vi "ois_ttc_merging.vi"() -> ()   [LabVIEW 2012]
uses:
  <vilib>/vision/Image Controls.llb/IMAQ Image.ctl
  <vilib>/picture/picture.llb/imagedata.ctl
  <vilib>/Utility/file.llb/Write To Spreadsheet File (DBL).vi
  <vilib>/vision/NI_Vision_Development_Module.lvlib
panel:
  in  "Tab Control":T1(tab)
  out "avi image with mask":T2(plugin-control)
  in  "video file":path=path "\\\\IFMB-02-024B-10\\Ischemia2/OOS/2019-05-29/2019-05-29_11-14-53.avi"
  in  "Use mask":bool=TRUE
  out "avi image":T2(plugin-control)
  in  "Range":cluster{"Lower value":sgl, "Upper value":sgl}={"Lower value"=103.29114, "Upper value"=255.0} {"Upper value" scale=0.0..255.0; "Lower value" scale=0.0..255.0}
  in  "IOS color":u32(colorbox)=16860
  in  "line color":u32(colorbox)=16711680
  in  "line Width":u32=1
  in  "TTC file":path=path "D:/Neurolab/ialdev/Ischemia YG/analisys/TTC images and OIS comparison/template/cortex_ttc_template.tif"
  in  "TTC Angle":dbl(knob) caption="Angle"
  in  "TTC Zoom":dbl(slide)=0.23059004545211792 caption="Zoom" scale=0.001..1.0
  in  "center X":u32(slide)=640 scale=0.0..640.0
  in  "center Y":u32(slide)=471
  in  "TTC horizontal reverse":bool caption="Horizontal reverse"
  in  "TTC vertical reverse":bool caption="Vertical reverse"
  out "front TTC image 2":T2(plugin-control) caption="TTC image"
  in  "Clear all points":bool
  out "XY Graph":cluster{dbl[], dbl[]}[](graph) caption="Saturation"
  in  "Add point":bool
  in  "Delete last point":bool
  in  "Save All Data":bool
  in  "filename":string="2019-05-29_11-14-53"
  in  "base path":path=path "\\\\IFMB-02-024B-10\\Ischemia2/OOS/2019-05-29"
  out "settings file":path=path "D:/Neurolab/ialdev/Ischemia YG/analisys/TTC images and OIS comparison/settings.ini"
  in  "Kernel Size (3,5,...)":i32=5 min=3 step=2
  in  "filtering":i32=5 min=0 max=100
  out "error out 2":errorcluster
  out "IOS borders and avi image":T3(array[cluster])
  out "ttc color on borders":cluster{"Slide":dbl, u32[]}[](array[cluster])
  out "IOS borders":u8[][](array[numeric])
  out "Array":dbl[](array[numeric])=[393.78881454467773, 286.3416109085083, 886.2111854553223, 655.6583890914917]
  out "ttc image data":T4={"image type"=0, "image depth"=24, "image"=array[143172 elements], "mask"=[], "colors"=[], "Rectangle"={"left"=0, "top"=0, "right"=246, "bottom"=194}}
  out "ios overlay":u32[][](array[numeric])
  out "error out 4":errorcluster
  out "dt":u32=2500
  in  "Time, min":dbl(slide)=2.057065217391304 scale=0.0..2.375
  out "error out":errorcluster
  out "TTC image in":T2
  in  "stop":bool=TRUE
  out "front TTC image":T2(plugin-control)
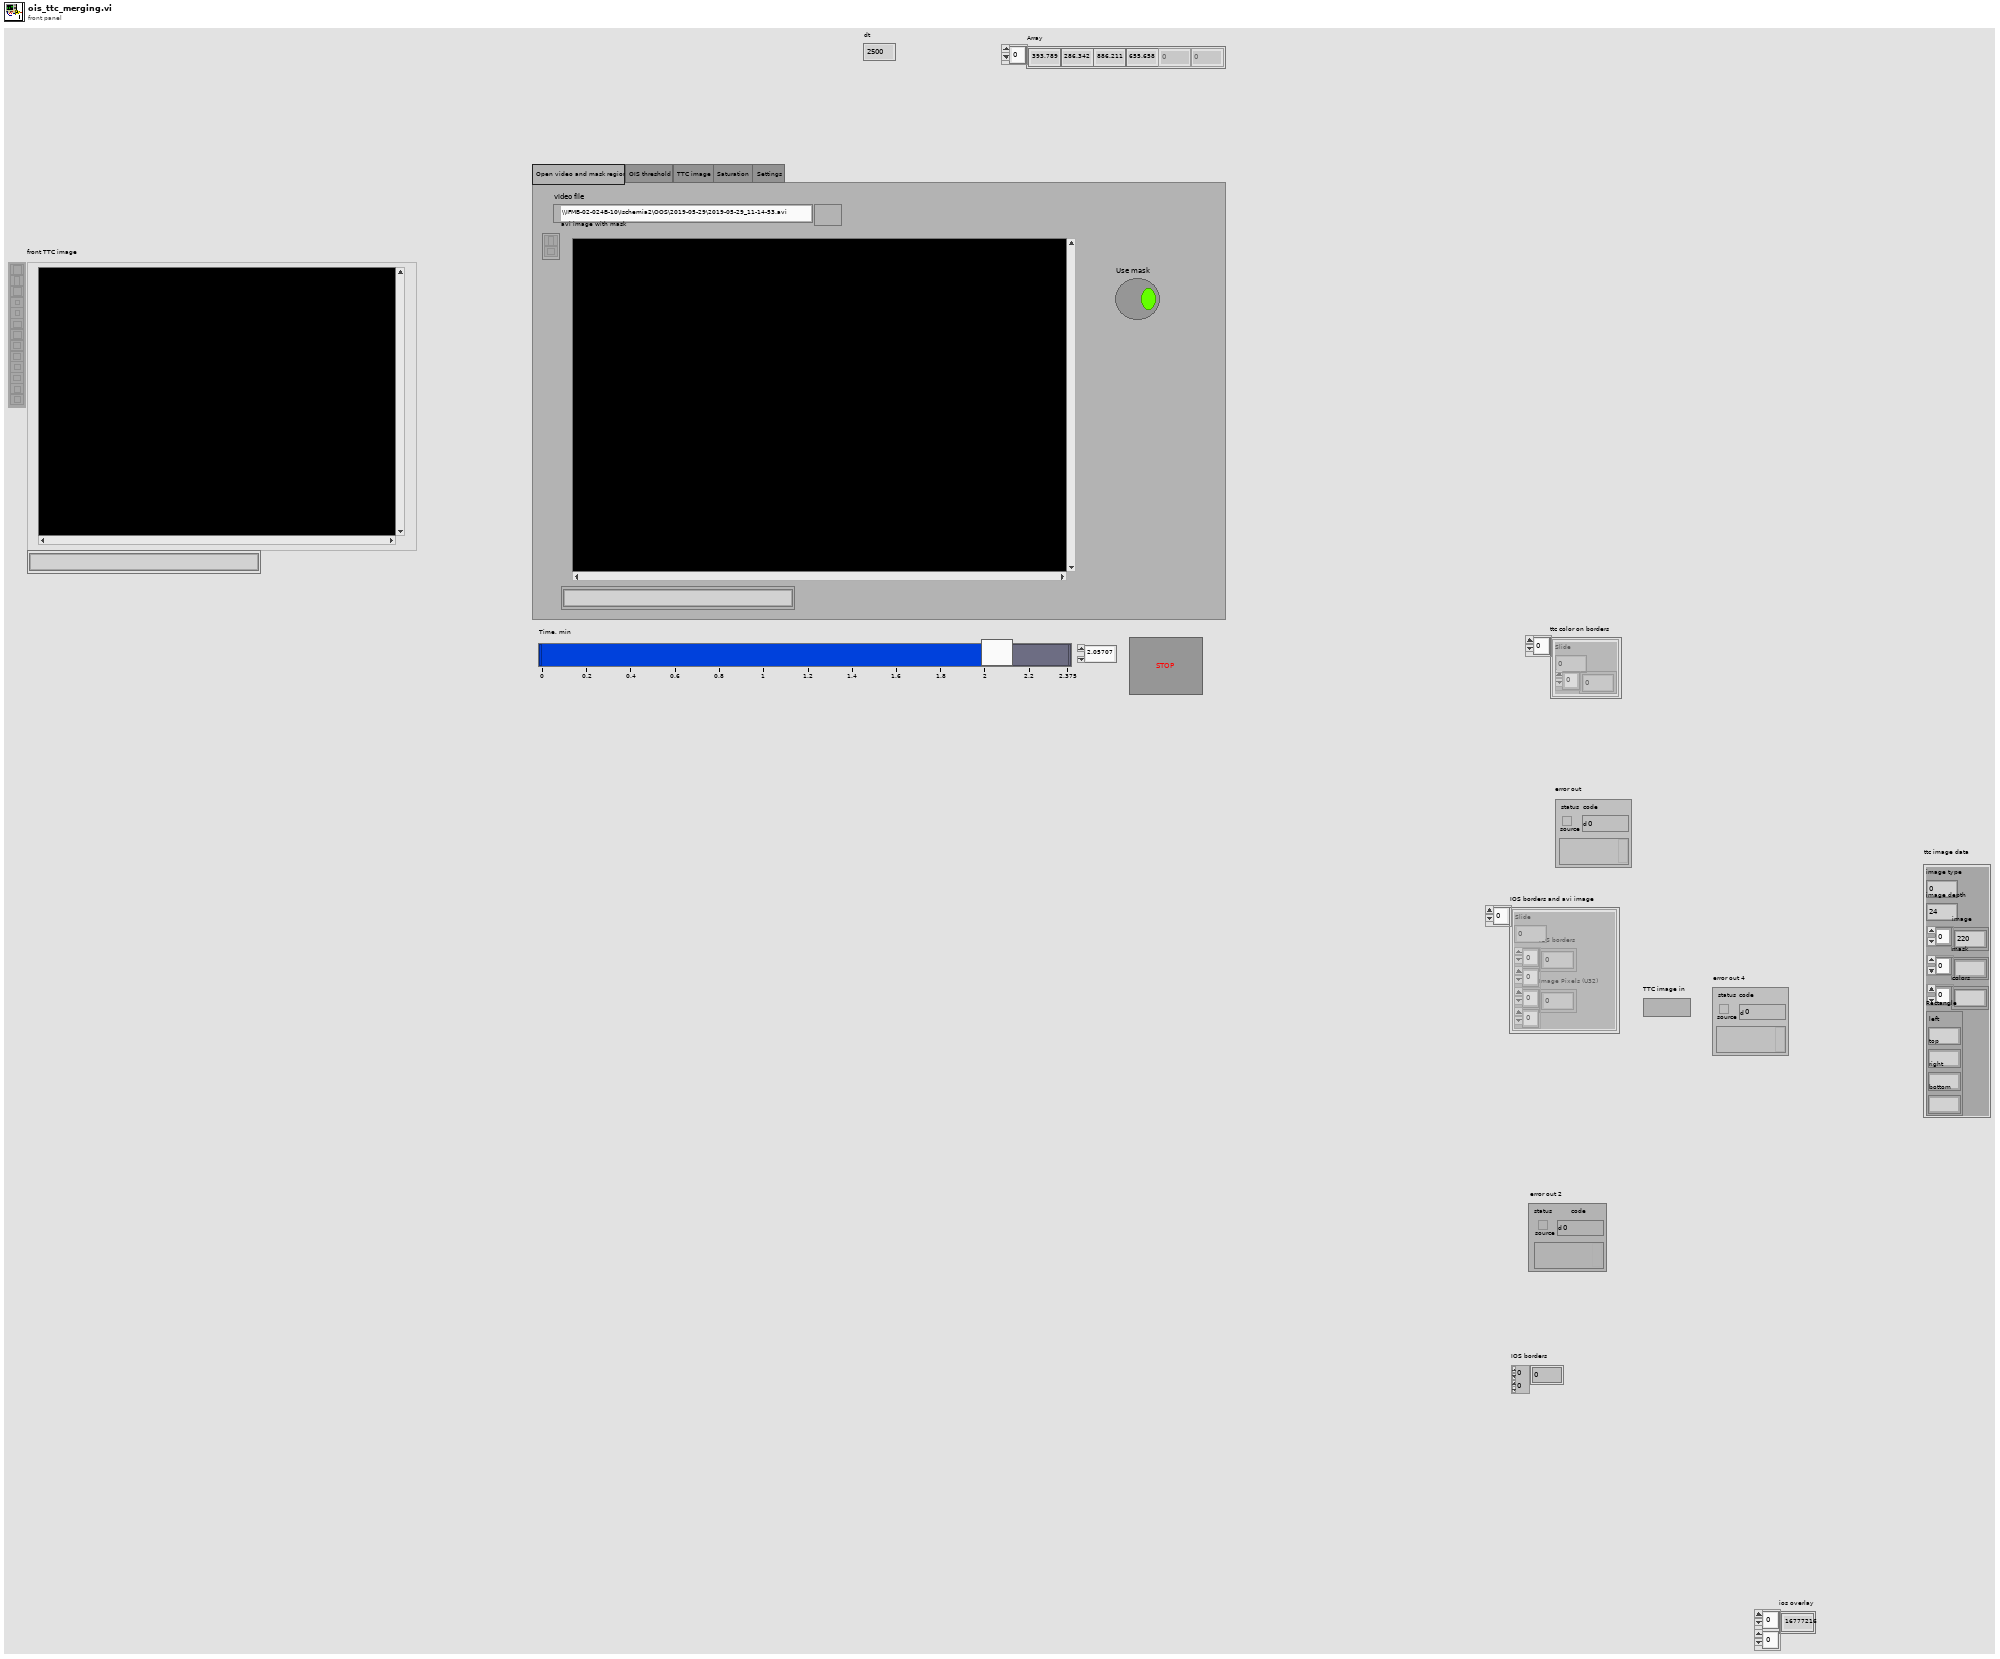
[diagram p1: front panel]
types:
  T1 = enum32{"Open video and mask region", "OIS threshold", "TTC image", "Saturation", "Settings"}
  T2 = typedef "IMAQ Image.ctl" = refnum<image>
  T3 = cluster{"Slide":dbl, "IOS borders":u8[][], "Image Pixels (U32)":u32[][]}[]
  T4 = typedef "imagedata.ctl" = cluster{"image type":i32, "image depth":i32, "image":u8[], "mask":u8[], "colors":u32[], "Rectangle":cluster{"left":i16, "top":i16, "right":i16, "bottom":i16}}
  T5 = typedef "Image Type" = u32
  T6 = enum16{"open", "replace", "create", "open or create", "replace or create", "replace or create with confirmation"}
  T7 = typedef "AviRefnum.ctl" = refnum<k1>
  T8 = cluster{"Range":cluster{"Lower value":sgl, "Upper value":sgl}, "IOS color":u32, "line color":u32, "line Width":u32}
  T9 = enum32{"AutoM", "Close", "Dilate", "Erode", "Gradient", "Gradient out", "Gradient in", "Hit miss", "Open", "PClose", "POpen", "Thick", "Thin"}
  T10 = cluster{"Global Rectangle":i32[], "Contours":cluster{"Contour Type":u32, "ROI Type":u32, "Points":i32[]}[]}
  T11 = cluster{"Time, min":dbl, "IOS borders":u8[][], "Image Pixels (U32)":u32[][]}
  T12 = cluster{"video file":path, "TTC file":path, "TTC Angle":dbl, "TTC Zoom":dbl, "center X":u32, "center Y":u32, "TTC horizontal reverse":bool, "TTC vertical reverse":bool, "ROI":cluster{"Global Rectangle":i32[], "Contours":cluster{"Contour Type":u32, "ROI Type":u32, "Points":i32[]}[]}, "Range":cluster{"Lower value":sgl, "Upper value":sgl}, "Image Pixels (U32)":u32[][], "ttc color on borders":cluster{"Slide":dbl, u32[]}[], "IOS borders and avi image":cluster{"Slide":dbl, "IOS borders":u8[][], "Image Pixels (U32)":u32[][]}[]}
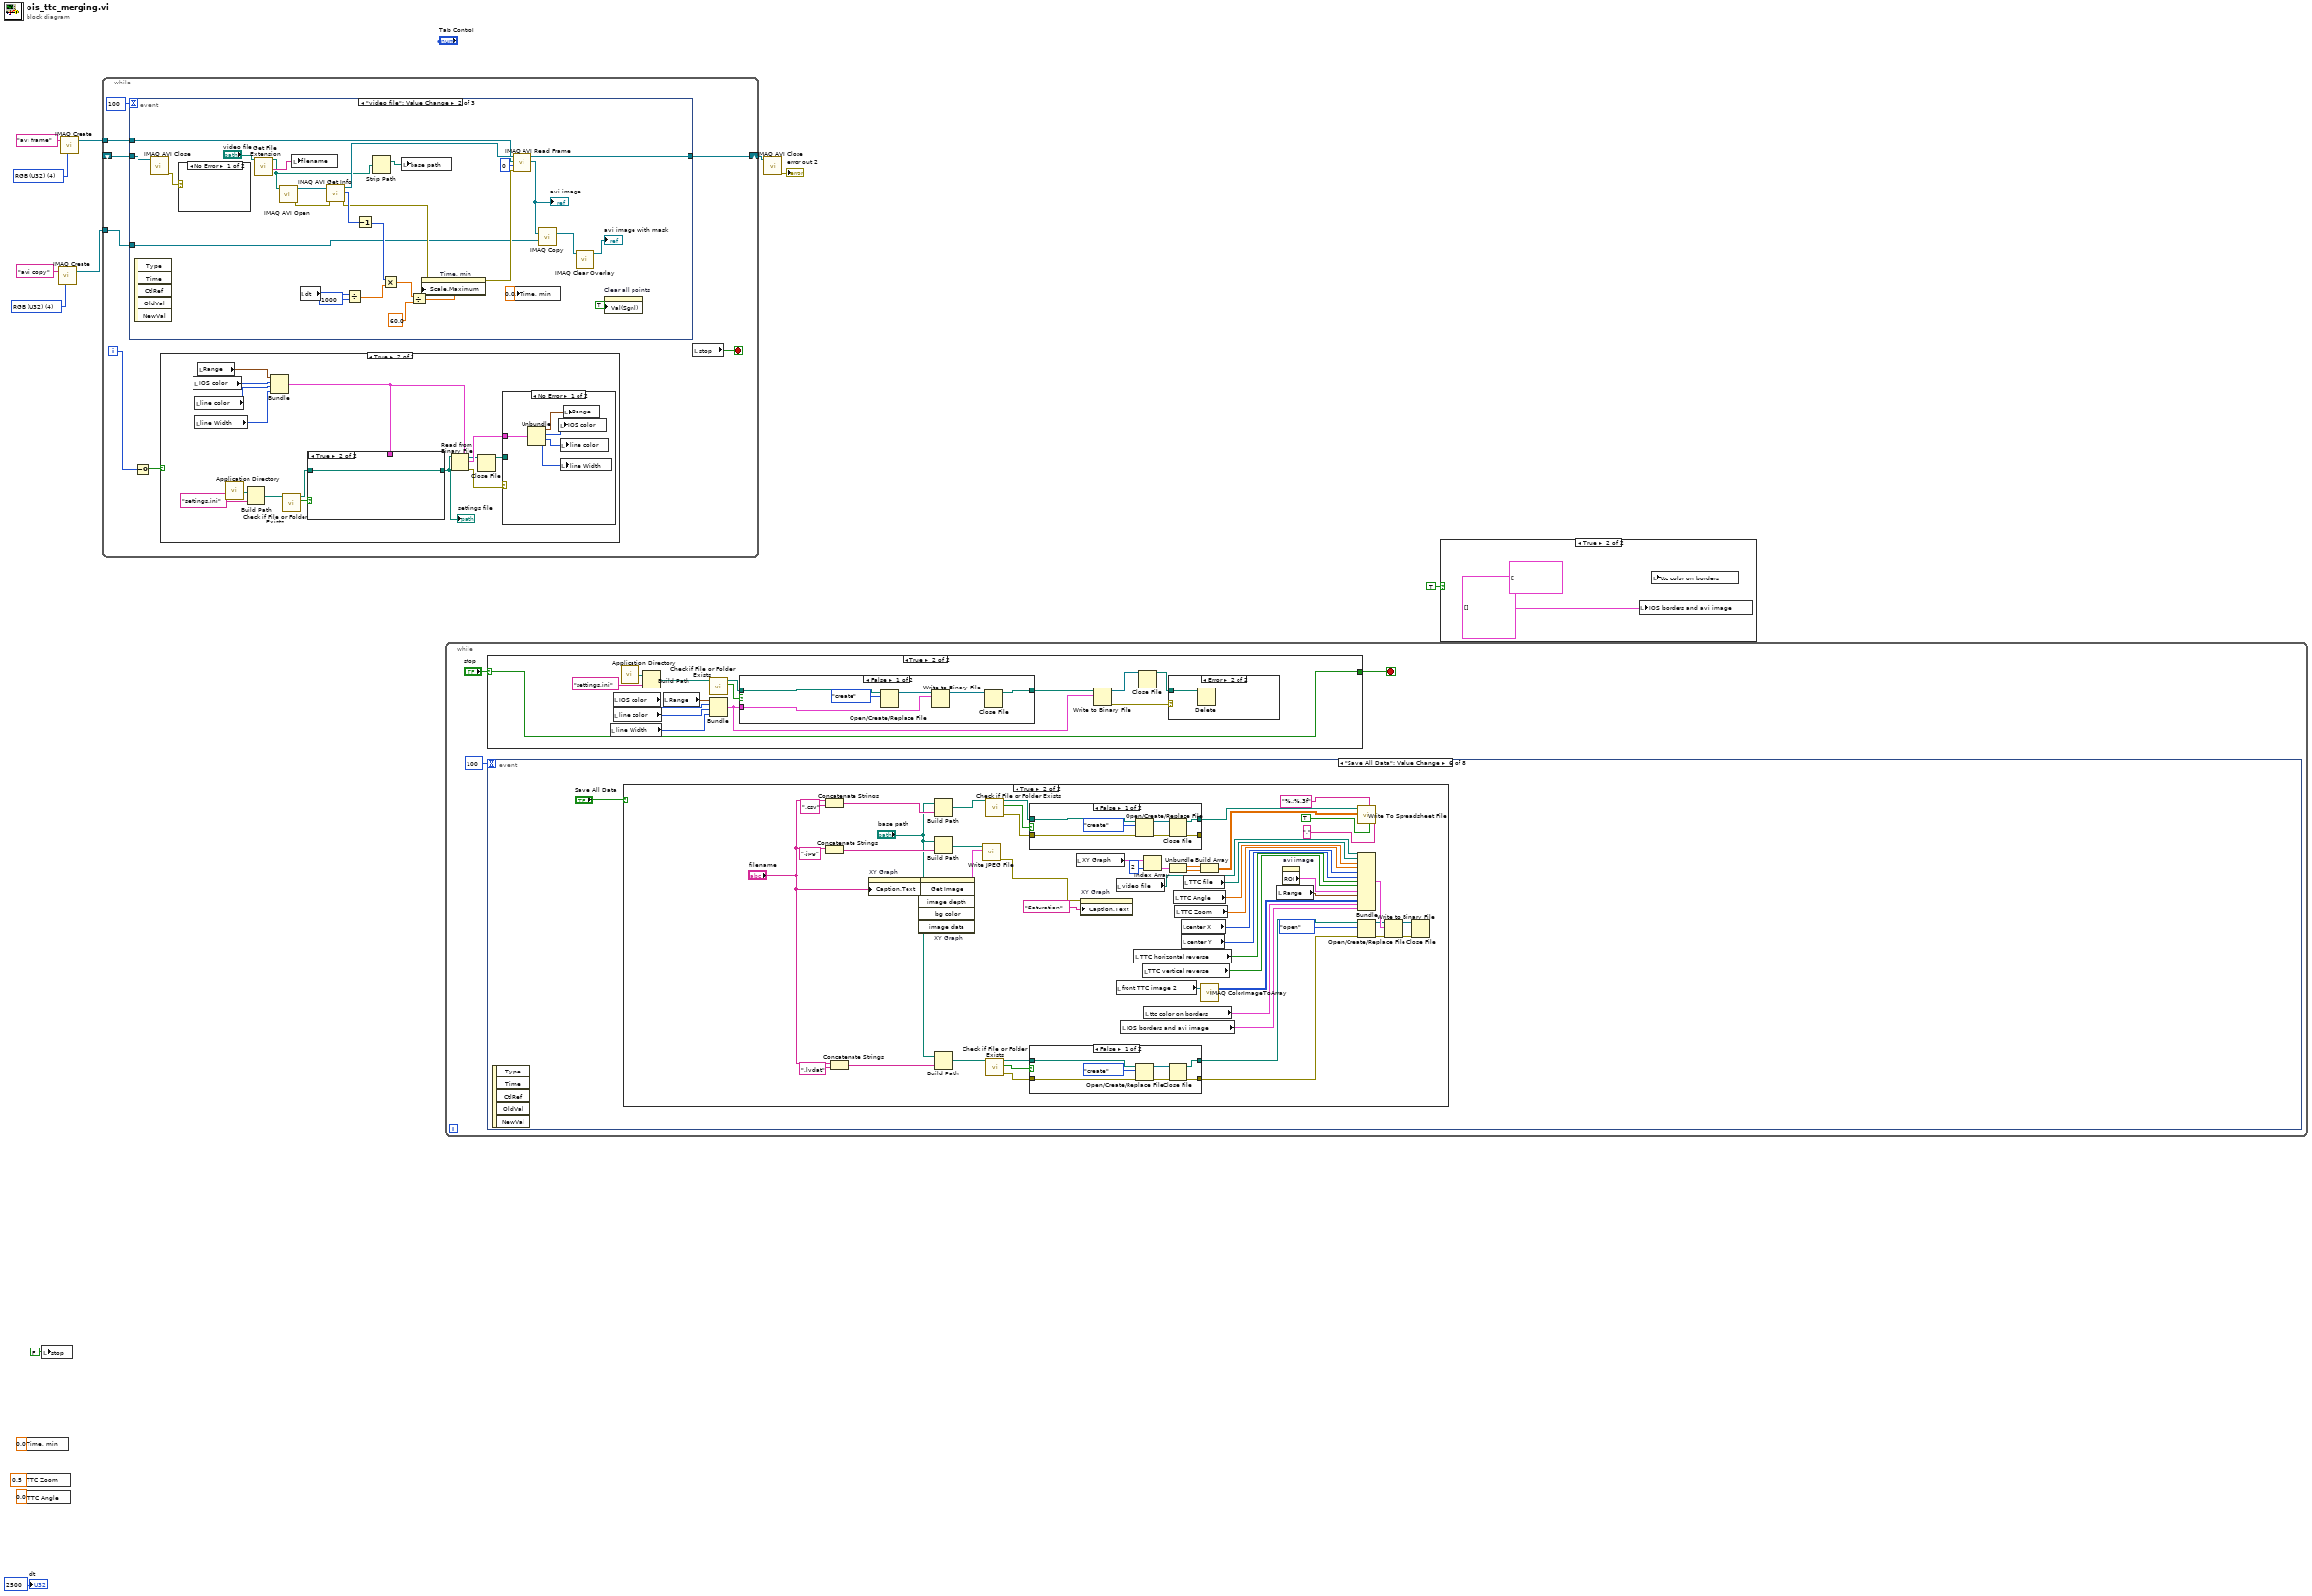
[diagram p0: block diagram]
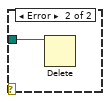
[diagram p4: hidden frame]
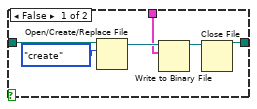
[diagram p5: hidden frame]
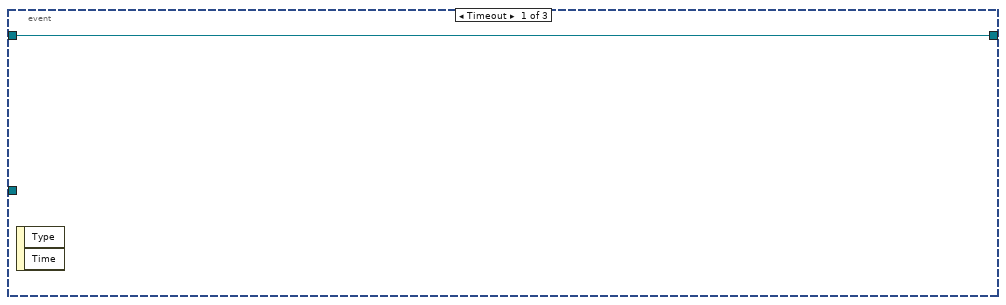
[diagram p6: hidden frame]
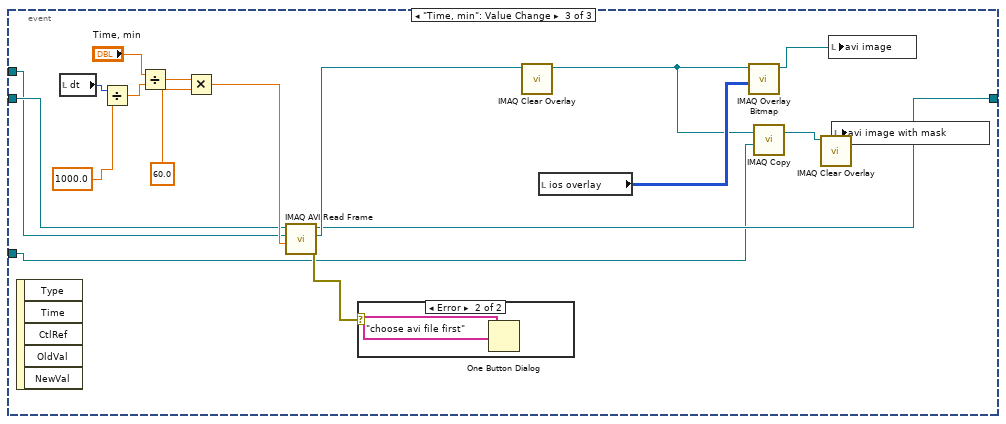
[diagram p8: hidden frame]
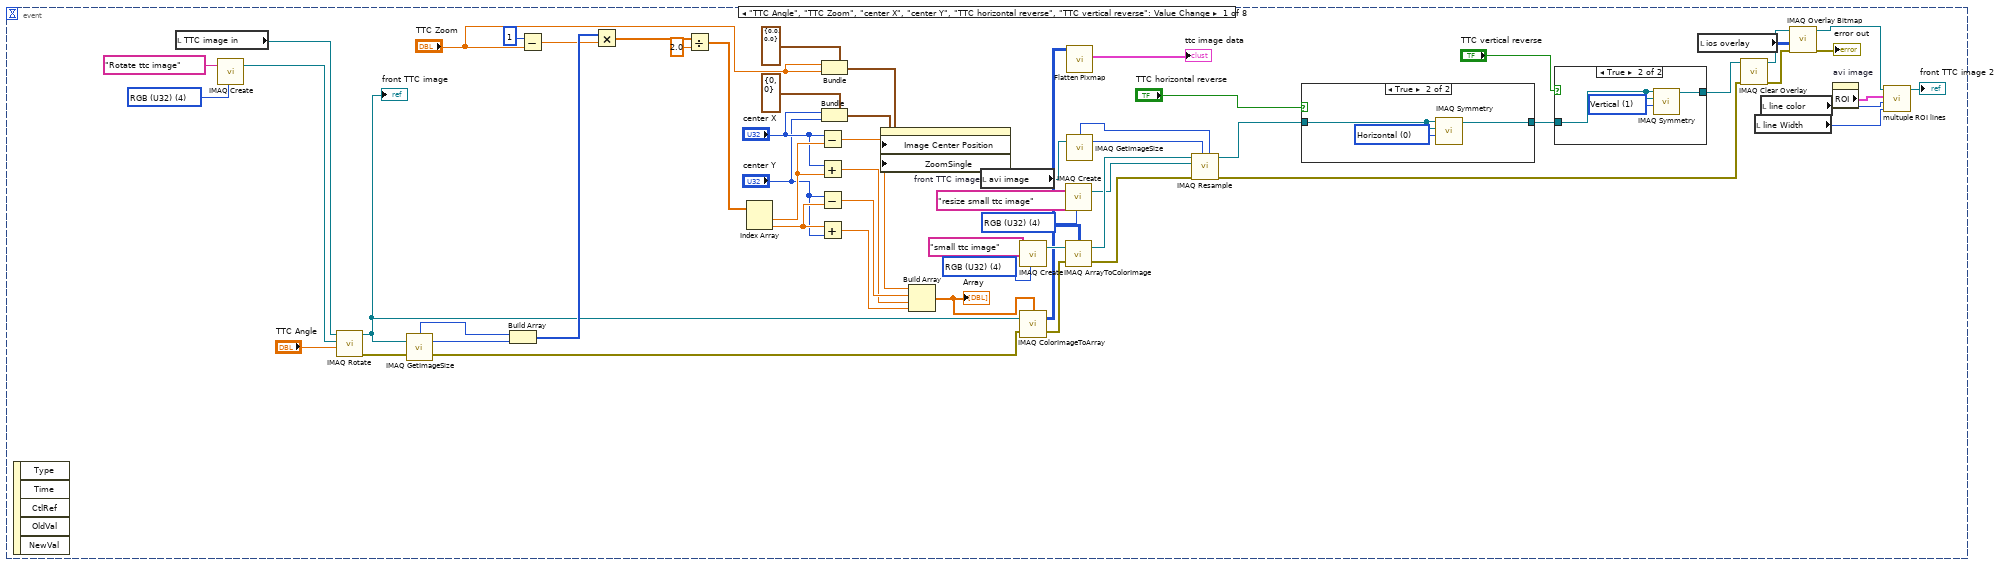
[diagram p13: hidden frame]
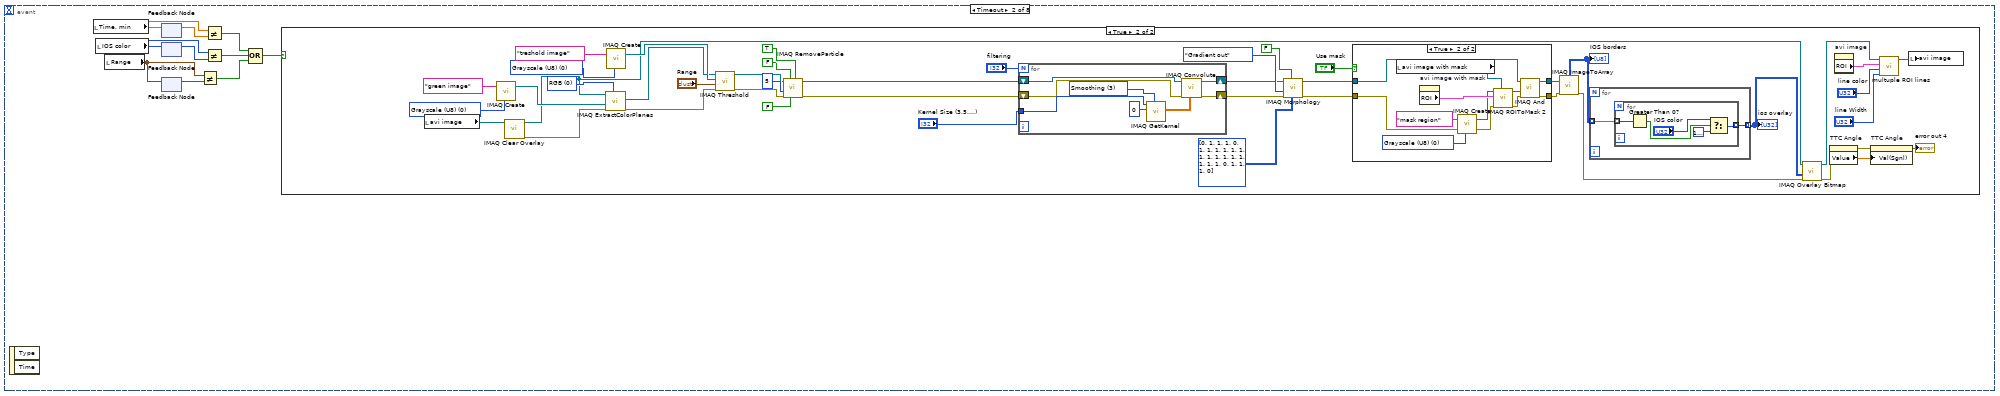
[diagram p16: hidden frame]
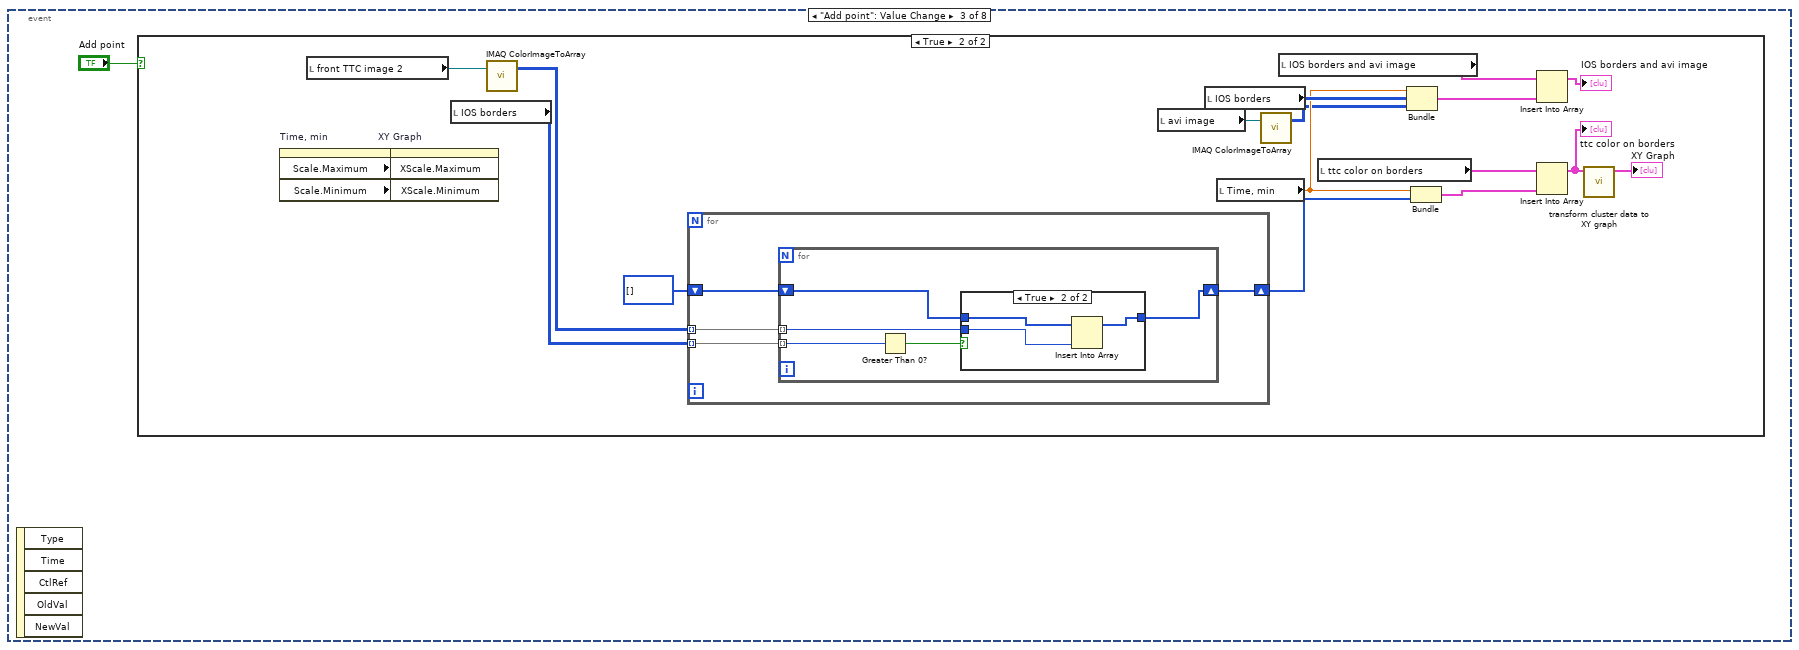
[diagram p19: hidden frame]
diagram:
  w2 = T5 4 items=["Grayscale (U8)", "Grayscale (I16)", "Grayscale (SGL)", "Complex (CSG)", "RGB (U32)", "HSL (U32)", "RGB (U64)", "Grayscale (U16)"] ("Image Type")
  w9 = T5 4 items=["Grayscale (U8)", "Grayscale (I16)", "Grayscale (SGL)", "Complex (CSG)", "RGB (U32)", "HSL (U32)", "RGB (U64)", "Grayscale (U16)"] ("Image Type")
  n1 = local write "Time, min"(0.0 ("Slide")) -> ()
  n2 = local write "TTC Zoom"(0.5 ("Zoom")) -> ()
  n3 = local write "TTC Angle"(0.0 ("Slide")) -> ()
  n4 = local write "stop"(FALSE ("stop")) -> ()
  n5 = call "IMAQ Create"("Image Name"="avi copy", "Image Type"=w2) -> ("New Image"=w1:T2)  [unwired: 3 in, 1 out]
  n6 = call "IMAQ Create"("Image Name"="avi frame", "Image Type"=w9) -> ("New Image"=w7:T2)  [unwired: 3 in, 1 out]
  n7 = while {
    shift-right: [w20] -> w6
    shift-left: _ -> [w18]
    tunnel: w7 -> [w19]
    tunnel: w1 -> [w17]
    i -> [w15]
    stop <- w22 stop-if-true
    n8 = event shown="[1] \"video file\": Value Change" {
      selector: _ -> [_ _ _]
      dyn-events: _ -> [_ _ _]
      timeout: 100 -> [_ _ _]
      tunnel: [w51 w64 w86] -> w20
      tunnel: w19 -> [_ w63 w84]
      tunnel: w18 -> [w51 w62 w85]
      tunnel: w17 -> [_ w58 w82]
      event Timeout {
        n9 = event-data() -> ()  [unwired: 1 in, 2 out]
      }
      event "video file": Value Change {
        n10 = event-data() -> ()  [unwired: 1 in, 5 out]
        n11 = call "IMAQ AVI Close"("Avi Refnum"=w62) -> ("error out"=w61:errorcluster)  [unwired: 10 in]
        n12 = case shown="No Error" w61 {
          frame No Error {
          }
          frame Error {
          }
        }
        n13 = call <vilib>:"Get File Extension.vi"("file"="video file") -> ("filename without extension"=w54:string, "dup file"=w53:path)  [unwired: 7 in, 2 out]
        n14 = call "IMAQ AVI Open"("AVI Path"=w53) -> ("error out"=w67:errorcluster, "Avi Refnum"=w79:T7)  [unwired: 9 in]
        n15 = local write "filename"(w54) -> ()
        n16 = local read "dt"() -> (w74:u32)
        n17 = call "IMAQ AVI Get Info"("error in (no error)"=w67, "Avi Refnum"=w79) -> ("error out"=w66:errorcluster, "Number of Frames"=w77:u32, "Avi Refnum (duplicate)"=w78:T7)  [unwired: 5 in, 2 out]
        n18 = Divide(x=w74, y=u32 1000) -> (x/y=w71:dbl)
        n19 = Decrement(x=w77) -> (x-1=w72:u32)
        n20 = Strip Path(path=w53) -> (stripped path=w52:path)  [unwired: 1 out]
        n21 = Multiply(x=w72, y=w71) -> (x*y=w70:dbl)
        n22 = local write "base path"(w52) -> ()
        n23 = Divide(x=w70, y=60.0) -> (x/y=w68:dbl)
        n24 = property on="Time, min" class="Slide (strict)"(error in=w66, "Scale.Maximum"=w68) -> (error out=w65:errorcluster)  [unwired: 1 in, 1 out]
        n25 = local write "Time, min"(0.0 ("Slide")) -> ()
        n26 = call "IMAQ AVI Read Frame"("error in (no error)"=w65, "Frame Number"=u32 0, "Image"=w63, "Avi Refnum"=w78) -> ("Image Out"=w59:T2, "Avi Refnum (duplicate)"=w64:T7)  [unwired: 4 in, 2 out]
        "avi image" <- w59
        n27 = call "IMAQ Copy"("Image Dst"=w58, "Image Src"=w59) -> ("Image Dst Out"=w57:T2)  [unwired: 4 in, 1 out]
        n28 = call "IMAQ Clear Overlay"("Image"=w57) -> ("Image Out"=→"avi image with mask":T2)  [unwired: 9 in, 1 out]
        n29 = property on="Clear all points" class="Bool (strict)"("Val(Sgnl)"=TRUE ("Value (Signaling)")) -> ()  [unwired: 2 in, 2 out]
      }
      event "Time, min": Value Change {
        n30 = event-data() -> ()  [unwired: 1 in, 5 out]
        n31 = local read "dt"() -> (w96:u32)
        n32 = Divide(x=w96, y=1000.0) -> (x/y=w93:dbl)
        n33 = Divide(x="Time, min", y=w93) -> (x/y=w92:dbl)
        n34 = Multiply(x=w92, y=60.0) -> (x*y=w90:dbl)
        n35 = call "IMAQ AVI Read Frame"("Frame Number"=w90, "Image"=w84, "Avi Refnum"=w85) -> ("error out"=w97:errorcluster, "Image Out"=w88:T2, "Avi Refnum (duplicate)"=w86:T7)  [unwired: 5 in, 1 out]
        n36 = case shown="Error" w97 {
          frame No Error {
          }
          frame Error {
            n37 = One Button Dialog(message="choose avi file first") -> ()  [unwired: 1 in, 1 out]
          }
        }
        n38 = call "IMAQ Clear Overlay"("Image"=w88) -> ("Image Out"=w81:T2)  [unwired: 9 in, 1 out]
        n39 = local read "ios overlay"() -> (w87:u32[][])
        n40 = call "IMAQ Overlay Bitmap"("Bitmap"=w87, "Image"=w81) -> ("Image Out"=w89:T2)  [unwired: 8 in, 1 out]
        n41 = call "IMAQ Copy"("Image Dst"=w82, "Image Src"=w81) -> ("Image Dst Out"=w83:T2)  [unwired: 4 in, 1 out]
        n42 = call "IMAQ Clear Overlay"("Image"=w83) -> ("Image Out"=w80:T2)  [unwired: 9 in, 1 out]
        n43 = local write "avi image"(w89) -> ()
        n44 = local write "avi image with mask"(w80) -> ()
      }
    }
    n45 = Equal To 0?(x=w15) -> (x = 0?=w16:bool)
    n46 = case shown="True" w16 {
      frame False {
      }
      frame True {
        n47 = local read "IOS color"() -> (w30:u32)
        n48 = local read "line color"() -> (w28:u32)
        n49 = local read "line Width"() -> (w29:u32)
        n50 = local read "Range"() -> (w31:cluster{"Lower value":sgl, "Upper value":sgl})
        n51 = call <vilib>:"Application Directory.vi"() -> ("Application Directory"=w37:path)
        n52 = Build Path(base path=w37, name or relative path="settings.ini") -> (appended path=w34:path)
        n53 = Bundle("Range"=w31, "IOS color"=w30, "line color"=w28, "line Width"=w29) -> (w27:T8)  [unwired: 1 in]
        n54 = call <vilib>:"Check if File or Folder Exists.vi"("path"=w34) -> ("file or folder exists?"=w35:bool, "dup path"=w36:path)  [unwired: 8 in, 1 out]
        n55 = case shown="True" w35 {
          tunnel: w36 -> [w49 w50]
          tunnel: [w44 w50] -> w32
          tunnel: w27 -> [w45 _]
          frame False {
            n56 = Open/Create/Replace File(file path (use dialog)=w49, operation (0:open)=T6."create") -> (refnum out=w47:refnum<file>)  [unwired: 4 in, 2 out]
            n57 = Write to Binary File(file (use dialog)=w47, data=w45) -> (refnum out=w46:refnum<file>)  [unwired: 4 in, 2 out]
            n58 = Close File(refnum=w46) -> (path=w44:path)  [unwired: 1 in, 1 out]
          }
          frame True {
          }
        }
        "settings file" <- w32
        n59 = Read from Binary File(5:w27, 11:w32) -> (0:w26:errorcluster, 2:w25:T8, 3:w24:refnum<file>)  [unwired: 4 in, 1 out]
        n60 = Close File(refnum=w24) -> (path=w23:path)  [unwired: 1 in, 1 out]
        n61 = case shown="No Error" w26 {
          tunnel: w25 -> [w38 _]
          tunnel: w23 -> [_ w43]
          frame No Error {
            n62 = Unbundle(w38) -> ("Range"=w39:cluster{"Lower value":sgl, "Upper value":sgl}, "IOS color"=w40:u32, "line color"=w41:u32, "line Width"=w42:u32)
            n63 = local write "IOS color"(w40) -> ()
            n64 = local write "line color"(w41) -> ()
            n65 = local write "line Width"(w42) -> ()
            n66 = local write "Range"(w39) -> ()
          }
          frame Error {
            n67 = Delete(path (use dialog)=w43) -> ()  [unwired: 4 in, 3 out]
          }
        }
      }
    }
    n68 = local read "stop"() -> (w22:bool)
  }
  n69 = while {
    stop <- w99 stop-if-true
    n70 = case shown="True" "stop" {
      selector: "stop" -> [w102 w117]
      tunnel: [w102 w117] -> w99
      frame False {
      }
      frame True {
        n71 = local read "line Width"() -> (w110:u32)
        n72 = local read "IOS color"() -> (w109:u32)
        n73 = local read "line color"() -> (w111:u32)
        n74 = call <vilib>:"Application Directory.vi"() -> ("Application Directory"=w103:path)
        n75 = Build Path(base path=w103, name or relative path="settings.ini") -> (appended path=w106:path)
        n76 = local read "Range"() -> (w108:cluster{"Lower value":sgl, "Upper value":sgl})
        n77 = call <vilib>:"Check if File or Folder Exists.vi"("path"=w106) -> ("file or folder exists?"=w105:bool, "dup path"=w104:path)  [unwired: 8 in, 1 out]
        n78 = Bundle("Range"=w108, "IOS color"=w109, "line color"=w111, "line Width"=w110) -> (w114:T8)  [unwired: 1 in]
        n79 = case shown="False" w105 {
          tunnel: w104 -> [w124 w125]
          tunnel: [w119 w125] -> w113
          tunnel: w114 -> [w120 _]
          frame False {
            n80 = Open/Create/Replace File(file path (use dialog)=w124, operation (0:open)=T6."create") -> (refnum out=w122:refnum<file>)  [unwired: 4 in, 2 out]
            n81 = Write to Binary File(file (use dialog)=w122, data=w120) -> (refnum out=w121:refnum<file>)  [unwired: 4 in, 2 out]
            n82 = Close File(refnum=w121) -> (path=w119:path)  [unwired: 1 in, 1 out]
          }
          frame True {
          }
        }
        n83 = Write to Binary File(file (use dialog)=w113, data=w114) -> (refnum out=w116:refnum<file>, error out=w115:errorcluster)  [unwired: 4 in, 1 out]
        n84 = Close File(refnum=w116) -> (path=w112:path)  [unwired: 1 in, 1 out]
        n85 = case shown="Error" w115 {
          tunnel: w112 -> [_ w118]
          frame No Error {
          }
          frame Error {
            n86 = Delete(path (use dialog)=w118) -> ()  [unwired: 4 in, 3 out]
          }
        }
      }
    }
    n87 = event shown="[5] \"Save All Data\": Value Change" {
      selector: _ -> [_ _ _ _ _ _ _ _]
      dyn-events: _ -> [_ _ _ _ _ _ _ _]
      timeout: 100 -> [_ _ _ _ _ _ _ _]
      event "TTC Angle", "TTC Zoom", "center X", "center Y", "TTC horizontal reverse", "TTC vertical reverse": Value Change {
        w150 = T5 4 items=["Grayscale (U8)", "Grayscale (I16)", "Grayscale (SGL)", "Complex (CSG)", "RGB (U32)", "HSL (U32)", "RGB (U64)", "Grayscale (U16)"] ("Image Type")
        w154 = T5 4 items=["Grayscale (U8)", "Grayscale (I16)", "Grayscale (SGL)", "Complex (CSG)", "RGB (U32)", "HSL (U32)", "RGB (U64)", "Grayscale (U16)"] ("Image Type")
        w183 = T5 4 items=["Grayscale (U8)", "Grayscale (I16)", "Grayscale (SGL)", "Complex (CSG)", "RGB (U32)", "HSL (U32)", "RGB (U64)", "Grayscale (U16)"] ("Image Type")
        n88 = event-data() -> ()  [unwired: 1 in, 5 out]
        n89 = local read "TTC image in"() -> (w148:T2)
        n90 = call "IMAQ Create"("Image Name"="Rotate ttc image", "Image Type"=w150) -> ("New Image"=w149:T2)  [unwired: 3 in, 1 out]
        n91 = call "IMAQ Rotate"("Angle (degrees)"="TTC Angle", "Image Dst"=w149, "Image Src"=w148) -> ("error out"=w132:errorcluster, "Image Dst Out"=w147:T2)  [unwired: 7 in]
        "front TTC image" <- w147
        n92 = call "IMAQ GetImageSize"("Image"=w147, "error in (no error)"=w132) -> ("Y Resolution"=w178:i32, "X Resolution"=w179:i32, "error out"=w131:errorcluster)  [unwired: 2 in]
        n93 = Build Array(w179, w178) -> (w170:i32[])
        n94 = Subtract(x=1, y="TTC Zoom") -> (x-y=w167:dbl)
        n95 = Multiply(x=w170, y=w167) -> (x*y=w169:dbl[])
        n96 = Divide(x=w169, y=2.0 ("Zoom")) -> (x/y=w166:dbl[])
        n97 = Index Array(array=w166) -> (element #1=w175:dbl, element #2=w174:dbl)  [unwired: 2 in]
        n98 = Subtract(x="center X", y=w175) -> (x-y=w176:dbl)
        n99 = Add(x="center X", y=w175) -> (x+y=w173:dbl)
        n100 = Subtract(x="center Y", y=w174) -> (x-y=w177:dbl)
        n101 = Add(x=w174, y="center Y") -> (x+y=w172:dbl)
        n102 = Bundle(cluster=cluster{"X":sgl, "Y":sgl} {"X"=0.0, "Y"=0.0} ("ZoomSingle:All Elements"), "X"="TTC Zoom", "Y"="TTC Zoom") -> (w162:cluster{"X":sgl, "Y":sgl})
        n103 = Bundle(cluster=cluster{"X":u32, "Y":u32} {"X"=0, "Y"=0} ("Center Position"), "X"="center X", "Y"="center Y") -> (w163:cluster{"X":u32, "Y":u32})
        n104 = property on="front TTC image" class="ImageControl"("Image Center Position"=w163, "ZoomSingle"=w162) -> ()  [unwired: 2 in, 2 out]
        n105 = Build Array(w176, w177, w173, w172) -> (w171:dbl[])
        "Array" <- w171
        n106 = local read "avi image"() -> (w157:T2)
        n107 = call "IMAQ Create"("Image Name"="small ttc image", "Image Type"=w183) -> ("New Image"=w182:T2)  [unwired: 3 in, 1 out]
        n108 = call "IMAQ ColorImageToArray"("Optional Rectangle"=w171, "Image"=w147, "error in (no error)"=w131) -> ("Image Pixels (U32)"=w181:u32[][], "error out"=w130:errorcluster)  [unwired: 1 in, 1 out]
        n109 = call "IMAQ Create"("Image Name"="resize small ttc image", "Image Type"=w154) -> ("New Image"=w152:T2)  [unwired: 3 in, 1 out]
        n110 = call "IMAQ ArrayToColorImage"("Image Pixels (U32)"=w181, "Image"=w182, "error in (no error)"=w130) -> ("Image Out"=w158:T2, "error out"=w129:errorcluster)  [unwired: 2 in]
        n111 = call <vilib>:"Flatten Pixmap.vi"("24-bit pixmap"=w181) -> ("image data"=→"ttc image data":T4)  [unwired: 10 in]
        n112 = call "IMAQ GetImageSize"("Image"=w157) -> ("Y Resolution"=w155:i32, "X Resolution"=w156:i32)  [unwired: 3 in, 1 out]
        n113 = call "IMAQ Resample"("X Resolution"=w156, "Y Resolution"=w155, "error in (no error)"=w129, "Image Dst"=w152, "Image Src"=w158) -> ("error out"=w128:errorcluster, "Image Dst Out"=w146:T2)  [unwired: 5 in]
        n114 = case shown="True" "TTC horizontal reverse" {
          tunnel: w146 -> [w189 w191]
          tunnel: [w189 w190] -> w145
          frame False {
          }
          frame True {
            w192 = u32 0 items=["Horizontal", "Vertical", "Central", "1st Diagonal", "2nd Diagonal"] ("Type of Symmetry")
            n115 = call "IMAQ Symmetry"("Type of Symmetry"=w192, "Image Dst"=w191, "Image Src"=w191) -> ("Image Dst Out"=w190:T2)  [unwired: 2 in, 1 out]
          }
        }
        n116 = case shown="True" "TTC vertical reverse" {
          tunnel: w145 -> [w185 w188]
          tunnel: [w185 w186] -> w133
          frame False {
          }
          frame True {
            w187 = u32 1 items=["Horizontal", "Vertical", "Central", "1st Diagonal", "2nd Diagonal"] ("Type of Symmetry")
            n117 = call "IMAQ Symmetry"("Type of Symmetry"=w187, "Image Dst"=w188, "Image Src"=w188) -> ("Image Dst Out"=w186:T2)  [unwired: 2 in, 1 out]
          }
        }
        n118 = local read "ios overlay"() -> (w160:u32[][])
        n119 = call "IMAQ Clear Overlay"("error in (no error)"=w128, "Image"=w133) -> ("error out"=w127:errorcluster, "Image Out"=w159:T2)  [unwired: 8 in]
        n120 = local read "line Width"() -> (w140:u32)
        n121 = local read "line color"() -> (w141:u32)
        n122 = call "IMAQ Overlay Bitmap"("error in (no error)"=w127, "Bitmap"=w160, "Image"=w159) -> ("error out"=→"error out":errorcluster, "Image Out"=w144:T2)  [unwired: 7 in]
        n123 = property on="avi image" class="ImageControl"() -> ("ROI"=w142:T10)  [unwired: 2 in, 2 out]
        n124 = call "multuple ROI lines.vi"("Width"=w140, "line color"=w141, "ROI"=w142, "Image in"=w144) -> ("Image out"=→"front TTC image 2":T2)  [unwired: 7 in]
      }
      event Timeout {
        n125 = event-data() -> ()  [unwired: 1 in, 2 out]
        n126 = local read "Time, min"() -> (w202:dbl)
        n127 = local read "IOS color"() -> (w199:u32)
        n128 = local read "Range"() -> (w197:cluster{"Lower value":sgl, "Upper value":sgl})
        n129 = feedback-in #1(w202) -> ()
        n130 = feedback #1() -> (w201:dbl)  [unwired: 1 in]
        n131 = feedback #2() -> (w200:u32)  [unwired: 1 in]
        n132 = feedback-in #2(w199) -> ()
        n133 = feedback #3() -> (w196:cluster{"Lower value":sgl, "Upper value":sgl})  [unwired: 1 in]
        n134 = feedback-in #3(w197) -> ()
        n135 = Not Equal?(x=w197, y=w196) -> (x != y?=w195:bool)
        n136 = Not Equal?(x=w202, y=w201) -> (x != y?=w194:bool)
        n137 = Not Equal?(x=w199, y=w200) -> (x != y?=w198:bool)
        n138 = Compound Arithmetic op=OR(w194, w198, w195) -> (w193:bool)
        n139 = case shown="True" w193 {
          frame False {
          }
          frame True {
            w243 = T5 0 items=["Grayscale (U8)", "Grayscale (I16)", "Grayscale (SGL)", "Complex (CSG)", "RGB (U32)", "HSL (U32)", "RGB (U64)", "Grayscale (U16)"] ("Image Type")
            w245 = u16 0 items=["RGB", "HSL", "HSV", "HSI"] ("Color Mode")
            w246 = T5 0 items=["Grayscale (U8)", "Grayscale (I16)", "Grayscale (SGL)", "Complex (CSG)", "RGB (U32)", "HSL (U32)", "RGB (U64)", "Grayscale (U16)"] ("Image Type")
            n140 = local read "avi image"() -> (w227:T2)
            n141 = call "IMAQ Create"("Image Name"="green image", "Image Type"=w246) -> ("New Image"=w244:T2)  [unwired: 3 in, 1 out]
            n142 = call "IMAQ Clear Overlay"("Image"=w227) -> ("error out"=w211:errorcluster, "Image Out"=w225:T2)  [unwired: 9 in]
            n143 = call "IMAQ ExtractColorPlanes"("Color Mode"=w245, "error in (no error)"=w211, "Green or Sat Plane"=w244, "Image Src"=w225) -> ("error out"=w210:errorcluster, "Green or Sat Plane out"=w226:T2)  [unwired: 4 in, 2 out]
            n144 = call "IMAQ Create"("Image Name"="treshold image", "Image Type"=w243) -> ("New Image"=w241:T2)  [unwired: 3 in, 1 out]
            n145 = call "IMAQ Threshold"("error in (no error)"=w210, "Range"="Range", "Image Dst"=w241, "Image Src"=w226) -> ("error out"=w234:errorcluster, "Image Dst Out"=w235:T2)  [unwired: 6 in]
            n146 = call "IMAQ RemoveParticle"("Connectivity 4/8 (8)"=TRUE, "Low Pass/High Pass (Low)"=FALSE, "Square/Hexa (Square)"=FALSE, "error in (no error)"=w234, "Number of Erosion"=5, "Image Src"=w235) -> ("error out"=w230:errorcluster, "Image Dst Out"=w231:T2)  [unwired: 1 in, 3 out]
            n147 = for {
              N: "filtering" -> [_]
              tunnel: "Kernel Size (3,5,...)" -> [w276]
              shift-right: [w272] -> w221
              shift-left: w231 -> [w271]
              shift-right: [w269] -> w220
              shift-left: w230 -> [w270]
              w274 = u16 3 items=["Gradient"=1, "Laplacian"=2, "Smoothing"=3, "Gaussian"=4] ("Kernel Family")
              n148 = call "IMAQ GetKernel"("Kernel Family"=w274, "Kernel Number"=0, "Kernel Size (3,5,...)"=w276) -> ("Kernel"=w273:sgl[][])  [unwired: 5 in, 3 out]
              n149 = call "IMAQ Convolute"("Kernel"=w273, "error in (no error)"=w270, "Image Src"=w271) -> ("error out"=w269:errorcluster, "Image Dst Out"=w272:T2)  [unwired: 7 in]
            }
            n150 = call "IMAQ Morphology"("Structuring Element"=i32[][] [[0, 1, 1, 1, 0], [1, 1, 1, 1, 1], [1, 1, 1, 1, 1], [1, 1, 1, 1, 1], [0, 1, 1, 1, 0]], "Square/Hexa (Square)"=FALSE, "error in (no error)"=w220, "Operation"=T9."Gradient out", "Image Src"=w221) -> ("error out"=w206:errorcluster, "Image Dst Out"=w207:T2)  [unwired: 2 in, 3 out]
            n151 = case shown="True" "Use mask" {
              tunnel: w207 -> [w249 w256]
              tunnel: w206 -> [w248 w251]
              tunnel: [w248 w254] -> w205
              tunnel: [w249 w253] -> w204
              frame False {
              }
              frame True {
                w258 = T5 0 items=["Grayscale (U8)", "Grayscale (I16)", "Grayscale (SGL)", "Complex (CSG)", "RGB (U32)", "HSL (U32)", "RGB (U64)", "Grayscale (U16)"] ("Image Type")
                n152 = local read "avi image with mask"() -> (w261:T2)
                n153 = property on="avi image with mask" class="ImageControl"() -> ("ROI"=w260:T10)  [unwired: 2 in, 2 out]
                n154 = call "IMAQ Create"("Image Name"="mask region", "Image Type"=w258, "error in (no error)"=w251) -> ("New Image"=w259:T2, "error out"=w252:errorcluster)  [unwired: 2 in]
                n155 = call "IMAQ ROIToMask 2"("Image Model"=w261, "error in (no error)"=w252, "ROI Descriptor"=w260, "Image"=w259) -> ("error out"=w250:errorcluster, "Image Out"=w255:T2)  [unwired: 5 in, 1 out]
                n156 = call "IMAQ And"("error in (no error)"=w250, "Image Src B"=w255, "Image Src A"=w256) -> ("error out"=w254:errorcluster, "Image Dst Out"=w253:T2)  [unwired: 7 in]
              }
            }
            n157 = call "IMAQ ImageToArray"("error in (no error)"=w205, "Image"=w204) -> ("error out"=w209:errorcluster, "Image Pixels (U8)"=w229:u8[][])  [unwired: 2 in, 3 out]
            "IOS borders" <- w229
            n158 = for {
              tunnel: w229 -> [w263] mode=indexing
              tunnel: [w262] -> w228 mode=indexing
              n159 = for {
                tunnel: w263 -> [w266] mode=indexing
                tunnel: [w264] -> w262 mode=indexing
                n160 = Greater Than 0?(x=w266) -> (x > 0?=w265:bool)
                n161 = Select(t="IOS color", s=w265, f=u32 16777216) -> (s? t:f=w264:u32)
              }
            }
            "ios overlay" <- w228
            n162 = call "IMAQ Overlay Bitmap"("error in (no error)"=w209, "Bitmap"=w228, "Image"=w225) -> ("error out"=w208:errorcluster, "Image Out"=w218:T2)  [unwired: 7 in]
            n163 = property on="TTC Angle" class="Knob (strict)"(error in=w208) -> (error out=w214:errorcluster, "Value"=w213:dbl)  [unwired: 1 in, 1 out]
            n164 = property on="avi image" class="ImageControl"() -> ("ROI"=w217:T10)  [unwired: 2 in, 2 out]
            n165 = property on="TTC Angle" class="Knob (strict)"(error in=w214, "Val(Sgnl)"=w213) -> (error out=→"error out 4":errorcluster)  [unwired: 1 in, 1 out]
            n166 = call "multuple ROI lines.vi"("Width"="line Width", "line color"="line color", "ROI"=w217, "Image in"=w218) -> ("Image out"=w219:T2)  [unwired: 7 in]
            n167 = local write "avi image"(w219) -> ()
          }
        }
      }
      event "Add point": Value Change {
        n168 = event-data() -> ()  [unwired: 1 in, 5 out]
        n169 = case shown="True" "Add point" {
          frame False {
          }
          frame True {
            n170 = property on="Time, min" class="Slide (strict)"() -> ("Scale.Maximum"=w291:dbl, "Scale.Minimum"=w292:dbl)  [unwired: 2 in, 2 out]
            n171 = local read "front TTC image 2"() -> (w294:T2)
            n172 = property on="XY Graph" class="XYGraph (strict)"("XScale.Maximum"=w291, "XScale.Minimum"=w292) -> ()  [unwired: 2 in, 2 out]
            n173 = local read "IOS borders"() -> (w295:u8[][])
            n174 = call "IMAQ ColorImageToArray"("Image"=w294) -> ("Image Pixels (U32)"=w285:u32[][])  [unwired: 3 in, 2 out]
            n175 = for {
              tunnel: w295 -> [w299] mode=indexing
              tunnel: w285 -> [w298] mode=indexing
              shift-right: [w297] -> w286
              shift-left: u32[] [] -> [w296]
              n176 = for {
                tunnel: w299 -> [w304] mode=indexing
                tunnel: w298 -> [w302] mode=indexing
                shift-right: [w301] -> w297
                shift-left: w296 -> [w300]
                n177 = Greater Than 0?(x=w304) -> (x > 0?=w303:bool)
                n178 = case shown="True" w303 {
                  tunnel: w302 -> [_ w308]
                  tunnel: [w305 w307] -> w301
                  tunnel: w300 -> [w305 w306]
                  frame False {
                  }
                  frame True {
                    n179 = Insert Into Array(array=w306, new element=w308) -> (w307:u32[])  [unwired: 1 in]
                  }
                }
              }
            }
            n180 = local read "avi image"() -> (w281:T2)
            n181 = local read "IOS borders"() -> (w283:u8[][])
            n182 = local read "Time, min"() -> (w282:dbl)
            n183 = call "IMAQ ColorImageToArray"("Image"=w281) -> ("Image Pixels (U32)"=w280:u32[][])  [unwired: 3 in, 2 out]
            n184 = local read "IOS borders and avi image"() -> (w278:T3)
            n185 = local read "ttc color on borders"() -> (w289:cluster{"Slide":dbl, u32[]}[])
            n186 = Bundle("Time, min"=w282, "IOS borders"=w283, "Image Pixels (U32)"=w280) -> (w284:T11)  [unwired: 1 in]
            n187 = Bundle("Time, min"=w282, w286) -> (w290:cluster{"Time, min":dbl, u32[]})  [unwired: 1 in]
            n188 = Insert Into Array(array=w278, new element=w284) -> (→"IOS borders and avi image":T3)  [unwired: 1 in]
            n189 = Insert Into Array(array=w289, new element=w290) -> (w288:cluster{"Slide":dbl, u32[]}[])  [unwired: 1 in]
            "ttc color on borders" <- w288
            n190 = call "transform cluster data to XY graph.vi"("data cluster array"=w288) -> ("XY data"=→"XY Graph":cluster{dbl[], dbl[]}[])  [unwired: 10 in]
          }
        }
      }
      event "Delete last point": Value Change {
        n191 = event-data() -> ()  [unwired: 1 in, 5 out]
        n192 = case shown="True" "Delete last point" {
          frame False {
          }
          frame True {
            n193 = local read "ttc color on borders"() -> (w315:cluster{"Slide":dbl, u32[]}[])
            n194 = Array Size(array=w315) -> (size(s)=w316:i32)
            n195 = local read "IOS borders and avi image"() -> (w311:T3)
            n196 = Decrement(x=w316) -> (x-1=w312:i32)
            n197 = Delete From Array(array=w311, index=w312) -> (array with subset deleted=w310:T3)  [unwired: 1 in, 1 out]
            n198 = Delete From Array(array=w315, index=w312) -> (array with subset deleted=w313:cluster{"Slide":dbl, u32[]}[])  [unwired: 1 in, 1 out]
            n199 = local write "IOS borders and avi image"(w310) -> ()
            n200 = local write "ttc color on borders"(w313) -> ()
            n201 = call "transform cluster data to XY graph.vi"("data cluster array"=w313) -> ("XY data"=w314:cluster{dbl[], dbl[]}[])  [unwired: 10 in]
            n202 = local write "XY Graph"(w314) -> ()
          }
        }
      }
      event "Clear all points": Value Change {
        n203 = event-data() -> ()  [unwired: 1 in, 5 out]
        n204 = case shown="True" "Clear all points" {
          frame False {
          }
          frame True {
            n205 = local write "IOS borders and avi image"(T3 [] ("array w/ subset deleted")) -> ()
            n206 = local write "ttc color on borders"(cluster{"Slide":dbl, u32[]}[] [] ("array w/ subset deleted")) -> ()
            n207 = local write "XY Graph"(cluster{dbl[], dbl[]}[] [] ("XY Graph")) -> ()
            n208 = local write "Clear all points"(FALSE ("Clear all points")) -> ()
          }
        }
      }
      event "Save All Data": Value Change {
        n209 = event-data() -> ()  [unwired: 1 in, 5 out]
        n210 = case shown="True" "Save All Data" {
          frame False {
          }
          frame True {
            n211 = Concatenate Strings("filename", ".jpg" ("string")) -> (w331:string)
            n212 = Concatenate Strings("filename", ".csv" ("string")) -> (w346:string)
            n213 = Concatenate Strings("filename", ".lvdat" ("string")) -> (w349:string)
            n214 = property on="XY Graph" class="XYGraph (strict)"("Caption.Text"="filename") -> (error out=w327:errorcluster)  [unwired: 2 in, 1 out]
            n215 = invoke on="XY Graph" class="XYGraph (strict)" method="Get Image"(error in=w327) -> ("image data"=w329:T4)  [unwired: 5 in, 5 out]
            n216 = Build Path(base path="base path", name or relative path=w346) -> (appended path=w342:path)
            n217 = Build Path(base path="base path", name or relative path=w331) -> (appended path=w328:path)
            n218 = Build Path(base path="base path", name or relative path=w349) -> (appended path=w350:path)
            n219 = call <vilib>:"Write JPEG File.vi"("image data"=w329, "path to JPEG file"=w328) -> ("error out"=w326:errorcluster)  [unwired: 8 in, 1 out]
            n220 = call <vilib>:"Check if File or Folder Exists.vi"("path"=w342) -> ("error out"=w345:errorcluster, "file or folder exists?"=w344:bool, "dup path"=w343:path)  [unwired: 8 in]
            n221 = call <vilib>:"Check if File or Folder Exists.vi"("path"=w350) -> ("error out"=w353:errorcluster, "file or folder exists?"=w360:bool, "dup path"=w361:path)  [unwired: 8 in]
            n222 = case shown="False" w344 {
              tunnel: w343 -> [w380 w384]
              tunnel: [w379 w384] -> w341
              tunnel: w345 -> [w378 w383]
              tunnel: [w376 w383] -> _
              frame False {
                n223 = Open/Create/Replace File(file path (use dialog)=w380, error in=w378, operation (0:open)=T6."create") -> (refnum out=w381:refnum<file>, error out=w377:errorcluster)  [unwired: 3 in, 1 out]
                n224 = Close File(refnum=w381, error in=w377) -> (path=w379:path, error out=w376:errorcluster)
              }
              frame True {
              }
            }
            n225 = case shown="False" w360 {
              tunnel: w361 -> [w389 w393]
              tunnel: [w388 w393] -> w359
              tunnel: w353 -> [w387 w392]
              tunnel: [w385 w392] -> w352
              frame False {
                n226 = Open/Create/Replace File(file path (use dialog)=w389, error in=w387, operation (0:open)=T6."create") -> (refnum out=w390:refnum<file>, error out=w386:errorcluster)  [unwired: 3 in, 1 out]
                n227 = Close File(refnum=w390, error in=w386) -> (path=w388:path, error out=w385:errorcluster)
              }
              frame True {
              }
            }
            n228 = local read "XY Graph"() -> (w340:cluster{dbl[], dbl[]}[])
            n229 = property on="XY Graph" class="XYGraph (strict)"(error in=w326, "Caption.Text"="Saturation") -> ()  [unwired: 1 in, 2 out]
            n230 = local read "video file"() -> (w351:path)
            n231 = local read "front TTC image 2"() -> (w366:T2)
            n232 = local read "IOS borders and avi image"() -> (w363:T3)
            n233 = local read "TTC horizontal reverse"() -> (w373:bool)
            n234 = local read "TTC vertical reverse"() -> (w372:bool)
            n235 = Index Array(array=w340, index=2) -> (element=w338:cluster{dbl[], dbl[]})
            n236 = local read "ttc color on borders"() -> (w364:cluster{"Slide":dbl, u32[]}[])
            n237 = Unbundle(w338) -> (w337:dbl[], w336:dbl[])
            n238 = local read "TTC Angle"() -> (w368:dbl)
            n239 = local read "TTC Zoom"() -> (w369:dbl)
            n240 = local read "center X"() -> (w371:u32)
            n241 = local read "center Y"() -> (w370:u32)
            n242 = local read "TTC file"() -> (w367:path)
            n243 = Build Array(w337, w336) -> (w335:dbl[][])
            n244 = call "IMAQ ColorImageToArray"("Image"=w366) -> ("Image Pixels (U32)"=w365:u32[][])  [unwired: 3 in, 2 out]
            n245 = local read "Range"() -> (w375:cluster{"Lower value":sgl, "Upper value":sgl})
            n246 = property on="avi image" class="ImageControl"() -> ("ROI"=w374:T10)  [unwired: 2 in, 2 out]
            n247 = call-poly <vilib>:"Write To Spreadsheet File.vi"("delimiter (\\t)"="," ("delimiter (\\t)"), "transpose? (no:F)"=TRUE, "format (%.3f)"="%.;%.3f", "2D data"=w335, "file path (dialog if empty)"=w341) -> ()  [unwired: 3 in, 1 out]
            n248 = Bundle("video file"=w351, "TTC file"=w367, "TTC Angle"=w368, "TTC Zoom"=w369, "center X"=w371, "center Y"=w370, "TTC horizontal reverse"=w373, "TTC vertical reverse"=w372, "ROI"=w374, "Range"=w375, "Image Pixels (U32)"=w365, "ttc color on borders"=w364, "IOS borders and avi image"=w363) -> (w362:T12)  [unwired: 1 in]
            n249 = Open/Create/Replace File(file path (use dialog)=w359, error in=w352, operation (0:open)=T6."open") -> (refnum out=w357:refnum<file>, error out=w354:errorcluster)  [unwired: 3 in, 1 out]
            n250 = Write to Binary File(file (use dialog)=w357, data=w362, error in=w354) -> (refnum out=w355:refnum<file>, error out=w356:errorcluster)  [unwired: 3 in, 1 out]
            n251 = Close File(refnum=w355, error in=w356) -> ()  [unwired: 2 out]
          }
        }
      }
      event "Time, min": Value Change {
        n252 = event-data() -> ()  [unwired: 1 in, 5 out]
      }
      event "TTC file": Value Change {
        w407 = T5 4 items=["Grayscale (U8)", "Grayscale (I16)", "Grayscale (SGL)", "Complex (CSG)", "RGB (U32)", "HSL (U32)", "RGB (U64)", "Grayscale (U16)"] ("Image Type")
        n253 = event-data() -> ()  [unwired: 1 in, 5 out]
        n254 = property on="front TTC image" class="ImageControl"("Zoom to Fit Mode"=TRUE) -> (error out=w405:errorcluster)  [unwired: 2 in, 1 out]
        n255 = property on="TTC Angle" class="Knob (strict)"("Val(Sgnl)"=0.0 ("Value (Signaling)")) -> ()  [unwired: 2 in, 2 out]
        n256 = property on="front TTC image" class="ImageControl"(error in=w405) -> (error out=w402:errorcluster, "X Zoom"=w404:sgl)  [unwired: 1 in, 1 out]
        n257 = call "IMAQ Create"("Image Name"="TTC image", "Image Type"=w407) -> ("New Image"=w408:T2)  [unwired: 3 in, 1 out]
        n258 = local write "TTC Zoom"(w404) -> ()
        n259 = property on="front TTC image" class="ImageControl"(error in=w402, "Zoom to Fit Mode"=FALSE) -> (error out=w401:errorcluster)  [unwired: 1 in, 1 out]
        n260 = call "IMAQ ReadFile"("File Path"="TTC file", "Image"=w408) -> ("Image Out"=w397:T2)  [unwired: 5 in, 4 out]
        "TTC image in" <- w397
        n261 = property on="front TTC image" class="ImageControl"(error in=w401) -> ("Image Center Position"=w400:cluster{"X":u32, "Y":u32})  [unwired: 1 in, 2 out]
        n262 = call "IMAQ GetImageSize"("Image"=w397) -> ("Y Resolution"=w396:i32, "X Resolution"=w395:i32)  [unwired: 3 in, 1 out]
        n263 = property on="center X" class="Slide (strict)"("Scale.Maximum"=w395) -> ()  [unwired: 2 in, 2 out]
        n264 = property on="center Y" class="Slide (strict)"("Scale.Maximum"=w396) -> ()  [unwired: 2 in, 2 out]
        n265 = Unbundle(w400) -> ("X"=w399:u32, "Y"=w398:u32)
        n266 = local write "center X"(w399) -> ()
        n267 = local write "center Y"(w398) -> ()
      }
    }
  }
  n268 = call "IMAQ AVI Close"("Avi Refnum"=w6) -> ("error out"=→"error out 2":errorcluster)  [unwired: 10 in]
  n269 = case shown="True" TRUE {
    frame False {
    }
    frame True {
      n270 = local write "IOS borders and avi image"(T3 [] ("IOS borders and avi image")) -> ()
      n271 = local write "ttc color on borders"(cluster{"Slide":dbl, u32[]}[] [] ("data cluster array")) -> ()
    }
  }
  "dt" <- u32 2500 ("Slide")
